vi "Test Draw To Picture ARGB.vi"(8 "error in (no error)":errorcluster, 11 "Test Case in":refnum<class "Image.lvclass">) -> (0 "error out":errorcluster, 3 "Test Case Out":refnum<class "Image.lvclass">)   [LabVIEW 2020, in "g_ar_toolkit.test.lvlib" / "Image.lvclass"]
uses:
  Image.lvclass
  C:/Program Files (x86)/National Instruments/LabVIEW 2020/vi.lib/Astemes/LUnit/Test Case.lvclass
  g_ar_toolkit.common/Image Size (Integer).ctl
  g_ar_toolkit.image/Image Draw Offset.ctl
  <vilib>/Astemes/LUnit/Test Case.lvclass/Test Case.ctl
  4993e8ee-a06a-463a-9684-69129f64d5ce.vi
  g_ar_toolkit.image/Create Image.vi
  g_ar_toolkit.image/CreateEmptyImageARGB.vi
  g_ar_toolkit.image/Copy Array to Image.vi
  g_ar_toolkit.image/CopyArrayToImageARGB.vi
  g_ar_toolkit.image/DrawImageToPictureARGB.vi/8cd07b1b-062e-4fe4-9e87-2eb3dc89fe0e.vi
  <vilib>/Astemes/LUnit/Append Pass Result.vi
  <vilib>/Astemes/LUnit/Append Fail Result.vi
  <vilib>/Astemes/LUnit/Describe Comparison.vi
  <vilib>/Astemes/LUnit/Compare Variants.vi
  g_ar_toolkit.image/CreateEmptyImageARGB.vi/3321fa97-f432-4e1e-8db9-a0df79aed21b.vi
  g_ar_toolkit.image/CopyArrayToImageARGB.vi/26c70cee-9332-41f4-9755-08948a885cbe.vi
  <vilib>/Astemes/LUnit/Run In UI.vi
  <vilib>/Utility/error.llb/Clear Errors.vi
  g_ar_toolkit.image/ARGBColourToU32.vi
  g_ar_toolkit.common/Module Path.vi
  <vilib>/Utility/error.llb/Error Cluster From Error Code.vi
  <vilib>/Astemes/LUnit/Describe Variant.vi
  Image.lvclass/Image.ctl
  g_ar_toolkit.image/g_ar_toolkit.image.lvlib
  g_ar_toolkit.common/g_ar_toolkit.common.lvlib
panel:
  out "Actual":picture
  out "Expected":picture
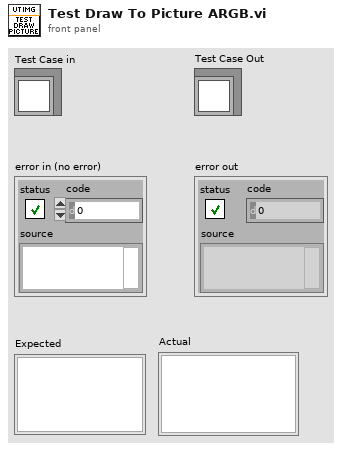
[diagram p1: front panel]
types:
  T1 = typedef "g_ar_toolkit.image.lvlib/Image Draw Offset.ctl" = cluster{"Left":i16, "Top":i16}
  T2 = typedef "g_ar_toolkit.common.lvlib/Image Size (Integer).ctl" = cluster{"Width":u16, "Height":u16}
  T3 = typedef "imagedata.ctl" = cluster{"image type":i32, "image depth":i32, "image":u8[], "mask":u8[], "colors":u32[], "Rectangle":cluster{"left":i16, "top":i16, "right":i16, "bottom":i16}}
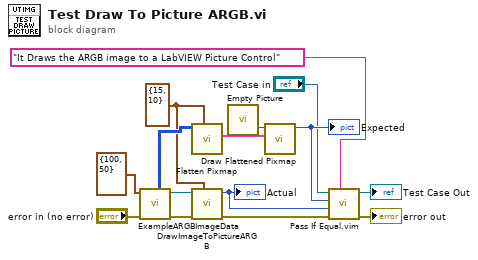
[diagram p0: block diagram]
diagram:
  w1 = T1 {"Left"=15, "Top"=10} ("Image Draw Offset (Default 0,0)")
  n1 = call "ExampleARGBImageData.vi"("error in (no error)"="error in (no error)", "Image Size"=T2 {"Width"=100, "Height"=50} ("Preallocated Image Size (Default - 0,0)")) -> ("error out"=w4:errorcluster, "Data Value Reference out"=w3:refnum<data-value>, "ARGB Array Data"=w2:u32[][])  [unwired: 6 in, 1 out]
  n2 = call <vilib>:"Flatten Pixmap.vi"("top left"=w1, "24-bit pixmap"=w2) -> ("image data"=w10:T3)  [unwired: 9 in]
  n3 = call "DrawImageToPictureARGB.vi"("Image Draw Offset (Default 0,0)"=w1, "error in (no error)"=w4, "ARGB Image Source"=w3) -> ("error out"=w11:errorcluster, "Picture"=w7:picture)  [unwired: 7 in]
  "Actual" <- w7
  n4 = call "Empty Picture"() -> ("empty picture"=w9:picture)
  n5 = call <vilib>:"Draw Flattened Pixmap.vi"("image data"=w10, "picture"=w9) -> ("new picture"=w8:picture)  [unwired: 7 in]
  "Expected" <- w8
  n6 = call "Pass If Equal.vim"("Description"="It Draws the ARGB image to a LabVIEW Picture Control", "error in (no error)"=w11, "Actual"=w7, "Expected"=w8, "LUnit Test Case In"="Test Case in") -> ("error out"=→"error out":errorcluster, "LUnit Test Case Out"=→"Test Case Out":refnum<class "Image.lvclass">)  [unwired: 5 in]
